vi "Stepper DAQ.vi"(8 "error in":errorcluster, 10 "semaphore":T1, 11 "BIBA 2017 Config":T8) -> (0 "error out":errorcluster, 2 "Timeout Counter":i32, 3 "Axis Data":T2)   [LabVIEW 2016, in "SMD-7615.lvlib"]
doc: "This VI reads Data (Digital Inputs, Motion I/O, Encoder Position & Velocity, ... ) of the specific Motor Device and publishes Data via corresponding Shared Variables."
uses:
  SMD-7615.lvlib
  CTL/Stepper Drive Config.ctl
  CTL/SV General.ctl
  CTL/SV Inputs.ctl
  CTL/SV Outputs.ctl
  CTL/Axis Data.ctl
  CTL/Motion IO.ctl
  CTL/Digital Lines (Read).ctl
  CTL/Status.ctl
  CTL/Encoder.ctl
  CTL/Position.ctl
  <vilib>/GPower/Error/Library/Append/AppendSingle.vi
  <vilib>/Utility/error.llb/Error Cluster From Error Code.vi
  <vilib>/ErrorRing/Error Ring.xnode
  <resource>/objmgr/nimcca.rc
  <vilib>/GPower/Error/GPError.lvlib
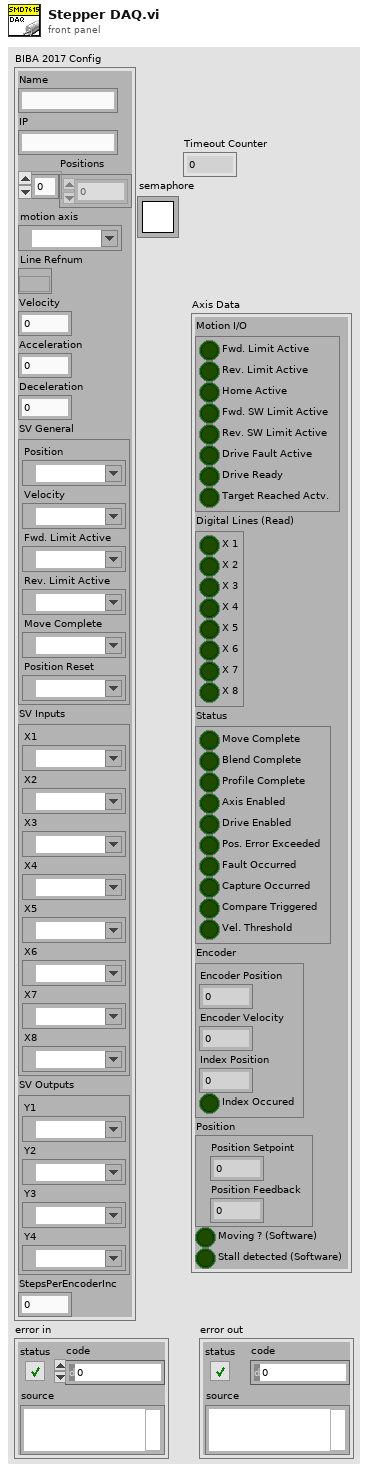
[diagram p1: front panel]
types:
  T1 = typedef "Semaphore RefNum" = refnum<k1>
  T2 = typedef "SMD-7615.lvlib/Axis Data.ctl" = cluster{"Motion I/O":T3, "Digital Lines (Read)":T4, "Status":T5, "Encoder":T6, "Position":T7, "Moving ? (Software)":bool, "Stall detected (Software)":bool}
  T3 = typedef "SMD-7615.lvlib/Motion IO.ctl" = cluster{"Fwd. Limit Active":bool, "Rev. Limit Active":bool, "Home Active":bool, "Fwd. SW Limit Active":bool, "Rev. SW Limit Active":bool, "Drive Fault Active":bool, "Drive Ready":bool, "Target Reached Actv.":bool}
  T4 = typedef "SMD-7615.lvlib/Digital Lines (Read).ctl" = cluster{"X 1":bool, "X 2":bool, "X 3":bool, "X 4":bool, "X 5":bool, "X 6":bool, "X 7":bool, "X 8":bool}
  T5 = typedef "SMD-7615.lvlib/Status.ctl" = cluster{"Move Complete":bool, "Blend Complete":bool, "Profile Complete":bool, "Axis Enabled":bool, "Drive Enabled":bool, "Pos. Error Exceeded":bool, "Fault Occurred":bool, "Capture Occurred":bool, "Compare Triggered":bool, "Vel. Threshold":bool}
  T6 = typedef "SMD-7615.lvlib/Encoder.ctl" = cluster{"Encoder Position":dbl, "Encoder Velocity":dbl, "Index Position":dbl, "Index Occured":bool}
  T7 = typedef "SMD-7615.lvlib/Position.ctl" = cluster{"Position Setpoint":dbl, "Position Feedback":dbl}
  T8 = typedef "SMD-7615.lvlib/Stepper Drive Config.ctl" = cluster{"Name":string, "IP":string, "Positions":dbl[], "motion axis ":refnum<k21>, "Line Refnum":refnum<k20>, "Velocity":dbl, "Acceleration":dbl, "Deceleration":dbl, "SV General":T9, "SV Inputs":T10, "SV Outputs":T11, "StepsPerEncoderInc":i32}
  T9 = typedef "SMD-7615.lvlib/SV General.ctl" = cluster{"Position":refnum<k21>, "Velocity":refnum<k21>, "Fwd. Limit Active":refnum<k21>, "Rev. Limit Active":refnum<k21>, "Move Complete":refnum<k21>, "Position Reset":refnum<k21>}
  T10 = typedef "SMD-7615.lvlib/SV Inputs.ctl" = cluster{"X1":refnum<k21>, "X2":refnum<k21>, "X3":refnum<k21>, "X4":refnum<k21>, "X5":refnum<k21>, "X6":refnum<k21>, "X7":refnum<k21>, "X8":refnum<k21>}
  T11 = typedef "SMD-7615.lvlib/SV Outputs.ctl" = cluster{"Y1":refnum<k21>, "Y2":refnum<k21>, "Y3":refnum<k21>, "Y4":refnum<k21>}
  T12 = cluster{"[0]":bool, "[1]":bool, "[2]":bool, "[3]":bool, "[4]":bool, "[5]":bool, "[6]":bool, "[7]":bool}
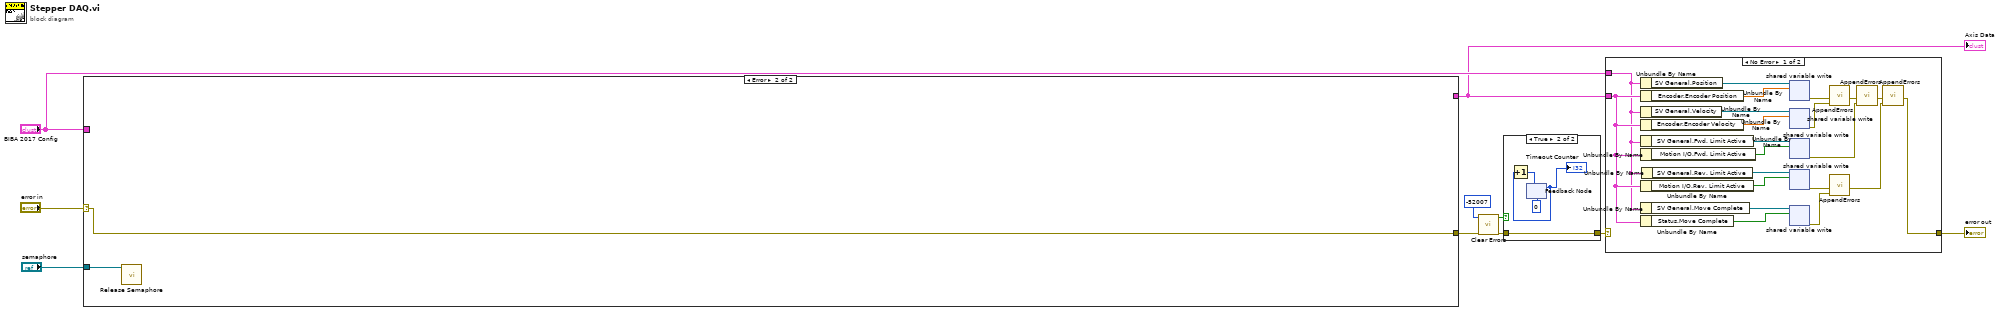
[diagram p0: block diagram]
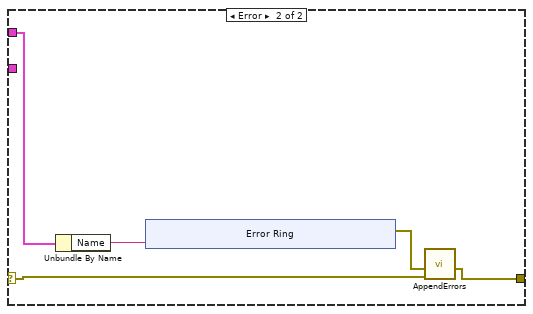
[diagram p3: hidden frame]
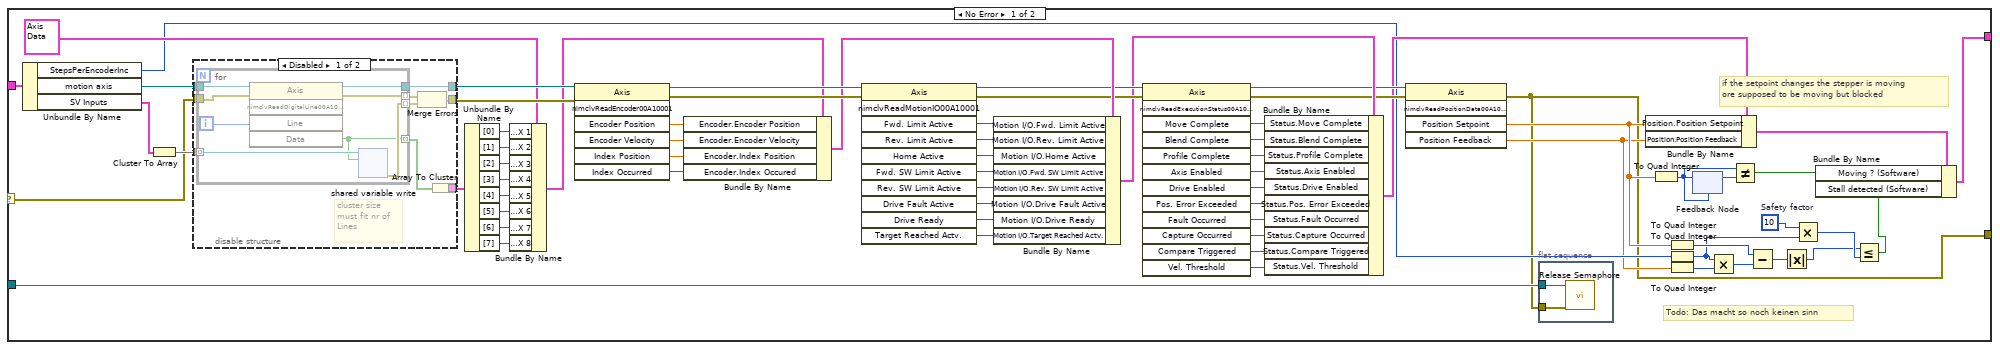
[diagram p4: hidden frame]
diagram:
  n1 = case shown="Error" "error in" {
    selector: "error in" -> [w70 w101]
    tunnel: [w11 w101] -> w7
    tunnel: "BIBA 2017 Config" -> [w71 _]
    tunnel: [w28 _] -> w4
    tunnel: "semaphore" -> [w12 w100]
    frame No Error {
      w16 = i64 10  # Safety factor
      # "Todo: Das macht so noch keinen sinn"
      # "if the setpoint changes the stepper is moving \nore supposed to be moving but blocked"
      n2 = Unbundle By Name(w71) -> ("StepsPerEncoderInc"=w24:i32, "motion axis"=w72:refnum<k21>, "SV Inputs"=w75:T10)
      n3 = Cluster To Array(cluster=w75) -> (array=w76:refnum<k21>[])
      n4 = disable-structure shown="Disabled" {
        disable-tunnel: w76 -> [w88 _]
        disable-tunnel: [w87 w98] -> w74
        disable-tunnel: [w85 w99] -> w73
        disable-tunnel: w72 -> [w84 w99]
        disable-tunnel: w70 -> [w83 w98]
        disable-tunnel: [w81 _] -> w69
        frame Disabled {
          # "cluster size\nmust fit nr of\nLines"
          n5 = for {
            tunnel: w83 -> [w96]
            tunnel: w84 -> [w97]
            tunnel: [w95] -> w85
            tunnel: [w93] -> w86 mode=indexing
            tunnel: w88 -> [w92] mode=indexing
            tunnel: [w91] -> w89 mode=indexing
            tunnel: [w90] -> w82 mode=indexing
            i -> [w94]
            n6 = invoke class="Axis" method="nimclvReadDigitalLine00A10001"(reference=w97, error in=w96, "Line"=w94) -> (reference out=w95:refnum<k21>, error out=w93:errorcluster, "Data"=w90:bool)  [unwired: 2 in, 2 out]
            n7 = shared-variable-write(w92, w90) -> (w91:errorcluster)  [unwired: 1 in, 1 out]
          }
          n8 = Merge Errors(w86, w89) -> (w87:errorcluster)
          n9 = Array To Cluster(array=w82) -> (cluster=w81:T12)
        }
        frame Enabled {
        }
      }
      n10 = Unbundle By Name(w69) -> ("[0]"=w67:bool, "[1]"=w65:bool, "[2]"=w64:bool, "[3]"=w63:bool, "[4]"=w62:bool, "[5]"=w61:bool, "[6]"=w60:bool, "[7]"=w59:bool)
      n11 = Bundle By Name(cluster=T2 {"Motion I/O"={"Fwd. Limit Active"=FALSE, "Rev. Limit Active"=FALSE, "Home Active"=FALSE, "Fwd. SW Limit Active"=FALSE, "Rev. SW Limit Active"=FALSE, "Drive Fault Active"=FALSE, "Drive Ready"=FALSE, "Target Reached Actv."=FALSE}, "Digital Lines (Read)"={"X 1"=FALSE, "X 2"=FALSE, "X 3"=FALSE, "X 4"=FALSE, "X 5"=FALSE, "X 6"=FALSE, "X 7"=FALSE, "X 8"=FALSE}, "Status"={"Move Complete"=FALSE, "Blend Complete"=FALSE, "Profile Complete"=FALSE, "Axis Enabled"=FALSE, "Drive Enabled"=FALSE, "Pos. Error Exceeded"=FALSE, "Fault Occurred"=FALSE, "Capture Occurred"=FALSE, "Compare Triggered"=FALSE, "Vel. Threshold"=FALSE}, "Encoder"={"Encoder Position"=0.0, "Encoder Velocity"=0.0, "Index Position"=0.0, "Index Occured"=FALSE}, "Position"={"Position Setpoint"=0.0, "Position Feedback"=0.0}, "Moving ? (Software)"=FALSE, "Stall detected (Software)"=FALSE} ("Axis Data"), "Digital Lines (Read).X 1"=w67, "Digital Lines (Read).X 2"=w65, "Digital Lines (Read).X 3"=w64, "Digital Lines (Read).X 4"=w63, "Digital Lines (Read).X 5"=w62, "Digital Lines (Read).X 6"=w61, "Digital Lines (Read).X 7"=w60, "Digital Lines (Read).X 8"=w59) -> (w66:T2)
      n12 = invoke class="Axis" method="nimclvReadEncoder00A10001"(reference=w73, error in=w74) -> (reference out=w77:refnum<k21>, error out=w78:errorcluster, "Encoder Position"=w58:dbl, "Encoder Velocity"=w57:dbl, "Index Position"=w56:dbl, "Index Occurred"=w55:bool)  [unwired: 5 in, 1 out]
      n13 = Bundle By Name(cluster=w66, "Encoder.Encoder Position"=w58, "Encoder.Encoder Velocity"=w57, "Encoder.Index Position"=w56, "Encoder.Index Occured"=w55) -> (w54:T2)
      n14 = invoke class="Axis" method="nimclvReadMotionIO00A10001"(reference=w77, error in=w78) -> (reference out=w45:refnum<k21>, error out=w44:errorcluster, "Fwd. Limit Active"=w53:bool, "Rev. Limit Active"=w52:bool, "Home Active"=w51:bool, "Fwd. SW Limit Active"=w50:bool, "Rev. SW Limit Active"=w49:bool, "Drive Fault Active"=w48:bool, "Drive Ready"=w47:bool, "Target Reached Actv."=w46:bool)  [unwired: 9 in, 1 out]
      n15 = Bundle By Name(cluster=w54, "Motion I/O.Fwd. Limit Active"=w53, "Motion I/O.Rev. Limit Active"=w52, "Motion I/O.Home Active"=w51, "Motion I/O.Fwd. SW Limit Active"=w50, "Motion I/O.Rev. SW Limit Active"=w49, "Motion I/O.Drive Fault Active"=w48, "Motion I/O.Drive Ready"=w47, "Motion I/O.Target Reached Actv."=w46) -> (w43:T2)
      n16 = invoke class="Axis" method="nimclvReadExecutionStatus00A10001"(reference=w45, error in=w44) -> (reference out=w31:refnum<k21>, error out=w32:errorcluster, "Move Complete"=w33:bool, "Blend Complete"=w34:bool, "Profile Complete"=w35:bool, "Axis Enabled"=w36:bool, "Drive Enabled"=w37:bool, "Pos. Error Exceeded"=w38:bool, "Fault Occurred"=w39:bool, "Capture Occurred"=w40:bool, "Compare Triggered"=w41:bool, "Vel. Threshold"=w42:bool)  [unwired: 11 in, 1 out]
      n17 = Bundle By Name(cluster=w43, "Status.Move Complete"=w33, "Status.Blend Complete"=w34, "Status.Profile Complete"=w35, "Status.Axis Enabled"=w36, "Status.Drive Enabled"=w37, "Status.Pos. Error Exceeded"=w38, "Status.Fault Occurred"=w39, "Status.Capture Occurred"=w40, "Status.Compare Triggered"=w41, "Status.Vel. Threshold"=w42) -> (w30:T2)
      n18 = invoke class="Axis" method="nimclvReadPositionData00A10001"(reference=w31, error in=w32) -> (error out=w11:errorcluster, "Position Setpoint"=w23:dbl, "Position Feedback"=w22:dbl)  [unwired: 3 in, 2 out]
      n19 = flat-sequence {
        tunnel: w12 -> [w80]
        tunnel: w11 -> [w79]
        frame #0 {
          n20 = call <vilib>:"Release Semaphore.vi"("error in (no error)"=w79, "semaphore"=w80) -> ()  [unwired: 4 in, 2 out]
        }
      }
      n21 = Bundle By Name(cluster=w30, "Position.Position Setpoint"=w23, "Position.Position Feedback"=w22) -> (w29:T2)
      n22 = To Quad Integer(1:w23) -> (0:w27:i64)
      n23 = To Quad Integer(1:w23) -> (0:w18:i64)
      n24 = To Quad Integer(1:w24) -> (0:w15:i64)
      n25 = To Quad Integer(1:w22) -> (0:w21:i64)
      n26 = feedback-in #1(w27) -> ()
      n27 = feedback #1(w27) -> (w25:i64)
      n28 = Multiply(x=w15, y=w21) -> (x*y=w20:i64)
      n29 = Not Equal?(x=w27, y=w25) -> (x != y?=w26:bool)
      n30 = Subtract(x=w18, y=w20) -> (x-y=w19:i64)
      n31 = Absolute Value(x=w19) -> (abs(x)=w13:i64)
      n32 = Multiply(x=w16, y=w15) -> (x*y=w14:i64)
      n33 = Less Or Equal?(x=w13, y=w14) -> (x <= y?=w17:bool)
      n34 = Bundle By Name(cluster=w29, "Moving ? (Software)"=w26, "Stall detected (Software)"=w17) -> (w28:T2)
    }
    frame Error {
      n35 = call <vilib>:"Release Semaphore.vi"("semaphore"=w100) -> ()  [unwired: 5 in, 2 out]
    }
  }
  "Axis Data" <- w4
  n36 = call <vilib>:"Clear Errors.vi"("error in (no error)"=w7, "specific error code to clear (0: all)"=-52007) -> ("error out"=w10:errorcluster, "specific error cleared?"=w9:bool)  [unwired: 4 in]
  n37 = case shown="True" w9 {
    tunnel: [w102 w103] -> w6
    tunnel: w10 -> [w102 w103]
    frame False {
    }
    frame True {
      n38 = feedback #2(0) -> (w104:i32)
      "Timeout Counter" <- w104
      n39 = Increment(x=w104) -> (x+1=w105:i32)
      n40 = feedback-in #2(w105) -> ()
    }
  }
  n41 = case shown="No Error" w6 {
    selector: w6 -> [_ w129]
    tunnel: [w107 w128] -> w3
    tunnel: "BIBA 2017 Config" -> [w108 w132]
    tunnel: w4 -> [w109 _]
    frame No Error {
      n42 = Unbundle By Name(w108) -> ("SV General.Position"=w110:refnum<k21>)
      n43 = Unbundle By Name(w109) -> ("Encoder.Encoder Position"=w111:dbl)
      n44 = Unbundle By Name(w108) -> ("SV General.Velocity"=w112:refnum<k21>)
      n45 = Unbundle By Name(w109) -> ("Encoder.Encoder Velocity"=w113:dbl)
      n46 = Unbundle By Name(w108) -> ("SV General.Fwd. Limit Active"=w114:refnum<k21>)
      n47 = Unbundle By Name(w109) -> ("Motion I/O.Fwd. Limit Active"=w115:bool)
      n48 = Unbundle By Name(w109) -> ("Motion I/O.Rev. Limit Active"=w117:bool)
      n49 = Unbundle By Name(w108) -> ("SV General.Move Complete"=w118:refnum<k21>)
      n50 = Unbundle By Name(w109) -> ("Status.Move Complete"=w119:bool)
      n51 = Unbundle By Name(w108) -> ("SV General.Rev. Limit Active"=w116:refnum<k21>)
      n52 = shared-variable-write(w110, w111) -> (w121:errorcluster)  [unwired: 1 in, 1 out]
      n53 = shared-variable-write(w112, w113) -> (w122:errorcluster)  [unwired: 1 in, 1 out]
      n54 = shared-variable-write(w114, w115) -> (w123:errorcluster)  [unwired: 1 in, 1 out]
      n55 = shared-variable-write(w116, w117) -> (w124:errorcluster)  [unwired: 1 in, 1 out]
      n56 = shared-variable-write(w118, w119) -> (w125:errorcluster)  [unwired: 1 in, 1 out]
      n57 = call-poly <vilib>:"AppendErrors.vi"("Error to append"=w122, "Error in"=w121) -> ("Appended errors out"=w120:errorcluster)  [unwired: 9 in]
      n58 = call-poly <vilib>:"AppendErrors.vi"("Error to append"=w125, "Error in"=w124) -> ("Appended errors out"=w127:errorcluster)  [unwired: 9 in]
      n59 = call-poly <vilib>:"AppendErrors.vi"("Error to append"=w123, "Error in"=w120) -> ("Appended errors out"=w126:errorcluster)  [unwired: 9 in]
      n60 = call-poly <vilib>:"AppendErrors.vi"("Error to append"=w127, "Error in"=w126) -> ("Appended errors out"=w107:errorcluster)  [unwired: 9 in]
    }
    frame Error {
      n61 = Unbundle By Name(w132) -> ("Name"=w131:string)
      n62 = xnode "Error Ring"("parameter 0"=w131) -> ("error out"=w130:errorcluster)
      n63 = call-poly <vilib>:"AppendErrors.vi"("Error to append"=w129, "Error in"=w130) -> ("Appended errors out"=w128:errorcluster)  [unwired: 9 in]
    }
  }
  "error out" <- w3
